vi "Lab Panel V6.00.vi"() -> ()   [LabVIEW 2017] (continued)
                              tunnel: w854 -> [_ _ _ w904 _]
                              tunnel: w853 -> [_ _ _ w914 _]
                              tunnel: w852 -> [_ _ _ w913 _]
                              tunnel: w851 -> [_ _ _ _ _]
                              tunnel: w850 -> [_ _ _ _ w920]
                              frame #0 {
                                w863 = "\\"
                                n604 = case shown="\"CHART TEST\", Default" w876 {
                                tunnel: ["L01-1-CHART TEST-" "L01-1-CYCLE TEST-" "L01-1-T-RISE TEST-"] -> w872
                                frame "CHART TEST", Default {
                                }
                                frame "CYCLE TEST" {
                                }
                                frame "T-RISE TEST" {
                                }
                                }
                                n605 = local read "SET LAB01-1"() -> (w871:T5)
                                n606 = Unbundle By Name(w871) -> ("DESCRIPTION"=w870:string)
                                n607 = Concatenate Strings(w866, "\\", w864, w863, w862, w863) -> (w873:string)
                                n608 = String To Path(string=w873) -> (path=w875:path)
                                n609 = Concatenate Strings(w873, w872, w870, "-", w869, ".tdms") -> (w861:string)
                                n610 = Create Folder(path (use dialog)=w875) -> (error out=w874:errorcluster)  [unwired: 2 in, 2 out]
                                n611 = call <vilib>:"Clear Errors.vi"("error in (no error)"=w874) -> ()  [unwired: 5 in, 2 out]
                                n612 = global write "Global 1.vi" "LAB01-1 FILE"(w861) -> ()
                              }
                              frame #1 {
                                (unwired) FALSE
                                n613 = String To Path(string=w882) -> (path=w880:path)
                                n614 = TDMS Open(6:FALSE, 10:T23."create or replace" ("operation (0:open)"), 11:w880) -> (0:w883:errorcluster, 3:→"TDMS LAB01-1":refnum<k34>)  [unwired: 4 in]
                              }
                              frame #2 {
                                n615 = local read "TDMS LAB01-1"() -> (w902:refnum<k34>)
                                n616 = local read "SET LAB01-1"() -> (w891:T5)
                                n617 = Build Array("Testers Name", "Description", "Set Test Cycles", "T-Rise minutes", "T-Rise Deg C") -> (w892:string[])
                                n618 = Unbundle(w891) -> ("NAME"=w890:string, "DESCRIPTION"=w889:string, "CYCLES"=w888:dbl, "T-RISE mins"=w887:dbl, "T-RISE deg C"=w886:dbl)
                                n619 = Number To Decimal String(number=w888) -> (decimal integer string=w901:string)  [unwired: 1 in]
                                n620 = Number To Decimal String(number=w887) -> (decimal integer string=w900:string)  [unwired: 1 in]
                                n621 = Number To Decimal String(number=w886) -> (decimal integer string=w899:string)  [unwired: 1 in]
                                n622 = Build Array(w890, w889, w901, w900, w899) -> (w898:string[])
                                n623 = TDMS Set Properties(5:w898, 7:w892, 11:w902) -> ()  [unwired: 3 in, 4 out]
                              }
                              frame #3 {
                                n624 = local read "DISP LAB01-1"() -> (w912:T4)
                                n625 = Concatenate Strings("LAB01-1  ", w904) -> (w903:string)
                                n626 = Two Button Dialog(message=w903, 1:w913, 2:w914) -> (T button?=w906:bool)
                                n627 = case shown="True" w906 {
                                tunnel: w912 -> [w917 w918]
                                tunnel: [w917 w918] -> w911
                                tunnel: [w916 w919] -> w910
                                tunnel: [w915 w919] -> w909
                                frame False {
                                n628 = Unbundle(w917) -> ("CYCLE"=w916:dbl, "MINS"=w915:dbl)  [unwired: 1 out]
                                }
                                frame True {
                                w919 = 0.0
                                }
                                }
                                n629 = Bundle(cluster=w911, "CYCLE"=w910, "MINS"=w909, "STATUS"="RUN") -> (w908:T4)
                                n630 = local write "DISP LAB01-1"(w908) -> ()
                              }
                              frame #4 {
                                n631 = local read "TEMP START LAB01-1"() -> (w922:cluster{"TL":dbl, "TN":dbl})
                                n632 = Bundle(cluster=w922, "TL"=w920, "TN"=w920) -> (w921:cluster{"TL":dbl, "TN":dbl})
                                n633 = local write "TEMP START LAB01-1"(w921) -> ()
                              }
                            }
                          }
                        }
                      }
                    }
                  }
                }
              }
              event "RUN LAB01-2": Value Change {
                n634 = event-data() -> ("NewVal"=w927:bool)  [unwired: 1 in, 5 out]
                n635 = local write "run lab01-2"(w927) -> ()
                n636 = case shown="True" w927 {
                  tunnel: w933 -> [_ w971]
                  tunnel: w932 -> [_ w970]
                  tunnel: w930 -> [w935 w969]
                  tunnel: w931 -> [_ w968]
                  tunnel: w929 -> [_ w967]
                  tunnel: [w934 w966] -> w928
                  tunnel: w926 -> [_ w965]
                  tunnel: w925 -> [_ w964]
                  tunnel: w924 -> [_ w963]
                  tunnel: w923 -> [_ w961]
                  frame False {
                    # "stop test"
                    n637 = stacked-sequence {
                      tunnel: w935 -> [w944 _]
                      tunnel: [w936 _] -> w934
                      frame #0 {
                        n638 = local read "DISP LAB01-2"() -> (w943:T4)
                        n639 = Unbundle(w943) -> ("CYCLE"=w941:dbl, "MINS"=w942:dbl)  [unwired: 1 out]
                        n640 = case shown="\"CHART TEST\", Default" w944 {
                          tunnel: w942 -> [_ _ w951]
                          tunnel: w941 -> [w949 w950 _]
                          tunnel: [w949 w950 w951] -> w940
                          frame "CHART TEST", Default {
                          }
                          frame "CYCLE TEST" {
                          }
                          frame "T-RISE TEST" {
                          }
                        }
                        n641 = local read "TDMS LAB01-2"() -> (w948:refnum<k34>)
                        n642 = Build Array("STOPPED") -> (w945:string[])
                        n643 = Build Array(w940) -> (w939:dbl[])
                        n644 = TDMS Write(0:w948, 5:"TEST RESULT", 7:w945, 9:w939) -> (4:w937:refnum<k34>, 15:w938:errorcluster)  [unwired: 2 in, 2 out]
                        n645 = TDMS Close(8:w938, 11:w937) -> (0:w936:errorcluster)  [unwired: 1 out]
                      }
                      frame #1 {
                        n646 = local read "DISP LAB01-2"() -> (w955:T4)
                        n647 = stacked-sequence {
                          tunnel: "LAB01-2" -> [w957 w959]
                          frame #0 {
                            n648 = call "sub vi - defrag tdms v1.vi"("panel id"=w957) -> ("error out"=w956:errorcluster)  [unwired: 10 in]
                            n649 = local write "data file error"(w956) -> ()
                          }
                          frame #1 {
                            n650 = call "Save data file (stop) v3.vi"("panel id"=w959) -> ("network file save error"=w958:errorcluster)  [unwired: 9 in, 1 out]
                            n651 = local write "RESULT LAB01-2"(FALSE) -> ()
                            n652 = local write "data file error"(w958) -> ()
                          }
                        }
                        n653 = Bundle(cluster=w955, "STATUS"="STOP") -> (w953:T4)  [unwired: 2 in]
                        n654 = local write "DISP LAB01-2"(w953) -> ()
                      }
                    }
                  }
                  frame True {
                    n655 = local read "SIG LAB01-2"() -> (w962:T2)
                    n656 = stacked-sequence {
                      seq-local: [w973 _] -> [_ w977]
                      tunnel: w971 -> [_ w987]
                      tunnel: w970 -> [_ w986]
                      tunnel: w969 -> [_ w985]
                      tunnel: w968 -> [_ w984]
                      tunnel: w967 -> [_ w983]
                      tunnel: [_ w982] -> w966
                      tunnel: w965 -> [_ w981]
                      tunnel: w964 -> [_ w980]
                      tunnel: w963 -> [_ w979]
                      tunnel: w962 -> [w972 w978]
                      tunnel: w961 -> [_ w976]
                      frame #0 {
                        n657 = Unbundle(w972) -> ("AMPS"=w975:dbl)  [unwired: 4 out]
                        n658 = call "Check For Amps on v1.vi"("ID"="LAB01-2", "amps"=w975) -> ("amps"=w973:bool)  [unwired: 9 in]
                      }
                      frame #1 {
                        n659 = case shown="True" w977 {
                          tunnel: w987 -> [_ w1000]
                          tunnel: w986 -> [_ w999]
                          tunnel: w985 -> [_ w998]
                          tunnel: w984 -> [_ w997]
                          tunnel: w983 -> [_ w996]
                          tunnel: [errorcluster {"status"=FALSE, "code"=0, "source"=""} ("error out") w995] -> w982
                          tunnel: w981 -> [_ w994]
                          tunnel: w980 -> [_ w993]
                          tunnel: w979 -> [_ w992]
                          tunnel: w978 -> [_ w991]
                          tunnel: w976 -> [_ w990]
                          frame False {
                            w988 = FALSE
                            n660 = local write "RUN LAB01-2"(w988) -> ()
                            n661 = local write "run lab01-2"(w988) -> ()
                          }
                          frame True {
                            n662 = stacked-sequence {
                              seq-local: [w1001 _ _ _ _] -> [_ w1025 _ _ _]
                              tunnel: w1000 -> [w1006 _ _ _ _]
                              tunnel: w999 -> [w1003 _ _ _ _]
                              tunnel: w998 -> [w1016 _ _ _ _]
                              tunnel: w997 -> [w1009 _ _ _ _]
                              tunnel: w996 -> [w1004 _ _ _ _]
                              tunnel: [_ w1020 _ _ _] -> w995
                              tunnel: w994 -> [_ _ _ w1047 _]
                              tunnel: w993 -> [_ _ _ w1046 _]
                              tunnel: w992 -> [_ _ _ w1045 _]
                              tunnel: w991 -> [_ _ _ _ _]
                              tunnel: w990 -> [_ _ _ _ w1060]
                              frame #0 {
                                w1002 = "\\"
                                n663 = local read "SET LAB01-2"() -> (w1011:T5)
                                n664 = case shown="\"CYCLE TEST\"" w1016 {
                                tunnel: ["L01-2-CHART TEST-" "L01-2-CYCLE TEST-" "L01-2-T-RISE TEST-"] -> w1012
                                frame "CHART TEST", Default {
                                }
                                frame "CYCLE TEST" {
                                }
                                frame "T-RISE TEST" {
                                }
                                }
                                n665 = Unbundle(w1011) -> ("DESCRIPTION"=w1010:string)  [unwired: 4 out]
                                n666 = Concatenate Strings(w1006, "\\", w1004, w1002, w1003, w1002) -> (w1013:string)
                                n667 = String To Path(string=w1013) -> (path=w1015:path)
                                n668 = Concatenate Strings(w1013, w1012, w1010, "-", w1009, ".tdms") -> (w1001:string)
                                n669 = Create Folder(path (use dialog)=w1015) -> (error out=w1014:errorcluster)  [unwired: 2 in, 2 out]
                                n670 = call <vilib>:"Clear Errors.vi"("error in (no error)"=w1014) -> ()  [unwired: 5 in, 2 out]
                                n671 = global write "Global 1.vi" "LAB01-2 FILE"(w1001) -> ()
                              }
                              frame #1 {
                                (unwired) FALSE
                                n672 = String To Path(string=w1025) -> (path=w1021:path)
                                n673 = TDMS Open(6:FALSE, 10:T23."create or replace" ("operation (0:open)"), 11:w1021) -> (0:w1020:errorcluster, 3:→"TDMS LAB01-2":refnum<k34>)  [unwired: 4 in]
                              }
                              frame #2 {
                                n674 = local read "SET LAB01-2"() -> (w1031:T5)
                                n675 = local read "TDMS LAB01-2"() -> (w1042:refnum<k34>)
                                n676 = Build Array("Testers Name", "Description", "Set Test Cycles", "T-Rise minutes", "T-Rise Deg C") -> (w1032:string[])
                                n677 = Unbundle(w1031) -> ("NAME"=w1030:string, "DESCRIPTION"=w1029:string, "CYCLES"=w1028:dbl, "T-RISE mins"=w1027:dbl, "T-RISE deg C"=w1026:dbl)
                                n678 = Number To Decimal String(number=w1028) -> (decimal integer string=w1041:string)  [unwired: 1 in]
                                n679 = Number To Decimal String(number=w1027) -> (decimal integer string=w1040:string)  [unwired: 1 in]
                                n680 = Number To Decimal String(number=w1026) -> (decimal integer string=w1039:string)  [unwired: 1 in]
                                n681 = Build Array(w1030, w1029, w1041, w1040, w1039) -> (w1038:string[])
                                n682 = TDMS Set Properties(5:w1038, 7:w1032, 11:w1042) -> ()  [unwired: 3 in, 4 out]
                              }
                              frame #3 {
                                n683 = local read "DISP LAB01-2"() -> (w1044:T4)
                                n684 = Concatenate Strings("LAB01-2  ", w1047) -> (w1048:string)
                                n685 = Two Button Dialog(message=w1048, 1:w1045, 2:w1046) -> (T button?=w1050:bool)
                                n686 = case shown="True" w1050 {
                                tunnel: w1044 -> [w1057 w1058]
                                tunnel: [w1057 w1058] -> w1054
                                tunnel: [w1056 w1059] -> w1053
                                tunnel: [w1055 w1059] -> w1052
                                frame False {
                                n687 = Unbundle(w1057) -> ("CYCLE"=w1056:dbl, "MINS"=w1055:dbl)  [unwired: 1 out]
                                }
                                frame True {
                                w1059 = 0.0
                                }
                                }
                                n688 = Bundle(cluster=w1054, "CYCLE"=w1053, "MINS"=w1052, "STATUS"="RUN") -> (w1043:T4)
                                n689 = local write "DISP LAB01-2"(w1043) -> ()
                              }
                              frame #4 {
                                n690 = local read "TEMP START LAB01-2"() -> (w1062:cluster{"TL":dbl, "TN":dbl})
                                n691 = Bundle(cluster=w1062, "TL"=w1060, "TN"=w1060) -> (w1061:cluster{"TL":dbl, "TN":dbl})
                                n692 = local write "TEMP START LAB01-2"(w1061) -> ()
                              }
                            }
                          }
                        }
                      }
                    }
                  }
                }
              }
              event "RUN LAB02-1": Value Change {
                n693 = event-data() -> ("NewVal"=w1068:bool)  [unwired: 1 in, 5 out]
                n694 = local read "SIG LAB02-1"() -> (w1064:T2)
                n695 = case shown="True" w1068 {
                  tunnel: w1074 -> [_ w1112]
                  tunnel: w1073 -> [_ w1111]
                  tunnel: w1071 -> [w1076 w1110]
                  tunnel: w1072 -> [_ w1109]
                  tunnel: w1070 -> [_ w1108]
                  tunnel: [w1075 w1107] -> w1069
                  tunnel: w1067 -> [_ w1106]
                  tunnel: w1066 -> [_ w1105]
                  tunnel: w1065 -> [_ w1104]
                  tunnel: w1064 -> [_ w1103]
                  tunnel: w1063 -> [_ w1102]
                  frame False {
                    # "stop test"
                    n696 = stacked-sequence {
                      tunnel: w1076 -> [w1085 _]
                      tunnel: [w1077 _] -> w1075
                      frame #0 {
                        n697 = local read "DISP LAB02-1"() -> (w1084:T4)
                        n698 = Unbundle(w1084) -> ("CYCLE"=w1082:dbl, "MINS"=w1083:dbl)  [unwired: 1 out]
                        n699 = case shown="\"CYCLE TEST\"" w1085 {
                          tunnel: w1083 -> [_ _ w1092]
                          tunnel: w1082 -> [w1090 w1091 _]
                          tunnel: [w1090 w1091 w1092] -> w1081
                          frame "CHART TEST", Default {
                          }
                          frame "CYCLE TEST" {
                          }
                          frame "T-RISE TEST" {
                          }
                        }
                        n700 = local read "TDMS LAB02-1"() -> (w1089:refnum<k34>)
                        n701 = Build Array("STOPPED") -> (w1086:string[])
                        n702 = Build Array(w1081) -> (w1080:dbl[])
                        n703 = TDMS Write(0:w1089, 5:"TEST RESULT", 7:w1086, 9:w1080) -> (4:w1078:refnum<k34>, 15:w1079:errorcluster)  [unwired: 2 in, 2 out]
                        n704 = TDMS Close(8:w1079, 11:w1078) -> (0:w1077:errorcluster)  [unwired: 1 out]
                      }
                      frame #1 {
                        n705 = local read "DISP LAB02-1"() -> (w1096:T4)
                        n706 = stacked-sequence {
                          tunnel: "LAB02-1" -> [w1098 w1100]
                          frame #0 {
                            n707 = call "sub vi - defrag tdms v1.vi"("panel id"=w1098) -> ("error out"=w1097:errorcluster)  [unwired: 10 in]
                            n708 = local write "data file error"(w1097) -> ()
                          }
                          frame #1 {
                            n709 = local write "RESULT LAB02-1"(FALSE) -> ()
                            n710 = call "Save data file (stop) v3.vi"("panel id"=w1100) -> ("network file save error"=w1099:errorcluster)  [unwired: 9 in, 1 out]
                            n711 = local write "data file error"(w1099) -> ()
                          }
                        }
                        n712 = Bundle(cluster=w1096, "STATUS"="STOP") -> (w1094:T4)  [unwired: 2 in]
                        n713 = local write "DISP LAB02-1"(w1094) -> ()
                      }
                    }
                  }
                  frame True {
                    n714 = stacked-sequence {
                      seq-local: [w1114 _] -> [_ w1118]
                      tunnel: w1112 -> [_ w1128]
                      tunnel: w1111 -> [_ w1127]
                      tunnel: w1110 -> [_ w1126]
                      tunnel: w1109 -> [_ w1125]
                      tunnel: w1108 -> [_ w1124]
                      tunnel: [_ w1123] -> w1107
                      tunnel: w1106 -> [_ w1122]
                      tunnel: w1105 -> [_ w1121]
                      tunnel: w1104 -> [_ w1120]
                      tunnel: w1103 -> [w1113 w1119]
                      tunnel: w1102 -> [_ w1117]
                      frame #0 {
                        n715 = Unbundle(w1113) -> ("AMPS"=w1116:dbl)  [unwired: 4 out]
                        n716 = call "Check For Amps on v1.vi"("ID"="LAB02-1", "amps"=w1116) -> ("amps"=w1114:bool)  [unwired: 9 in]
                      }
                      frame #1 {
                        n717 = case shown="True" w1118 {
                          tunnel: w1128 -> [_ w1141]
                          tunnel: w1127 -> [_ w1140]
                          tunnel: w1126 -> [_ w1139]
                          tunnel: w1125 -> [_ w1138]
                          tunnel: w1124 -> [_ w1137]
                          tunnel: [errorcluster {"status"=FALSE, "code"=0, "source"=""} ("error out") w1136] -> w1123
                          tunnel: w1122 -> [_ w1135]
                          tunnel: w1121 -> [_ w1134]
                          tunnel: w1120 -> [_ w1133]
                          tunnel: w1119 -> [_ w1132]
                          tunnel: w1117 -> [_ w1131]
                          frame False {
                            w1130 = FALSE
                            n718 = local write "RUN LAB02-1"(w1130) -> ()
                            n719 = local write "run lab02-1"(w1130) -> ()
                          }
                          frame True {
                            n720 = stacked-sequence {
                              seq-local: [w1142 _ _ _ _] -> [_ w1166 _ _ _]
                              tunnel: w1141 -> [w1147 _ _ _ _]
                              tunnel: w1140 -> [w1144 _ _ _ _]
                              tunnel: w1139 -> [w1157 _ _ _ _]
                              tunnel: w1138 -> [w1150 _ _ _ _]
                              tunnel: w1137 -> [w1145 _ _ _ _]
                              tunnel: [_ w1161 _ _ _] -> w1136
                              tunnel: w1135 -> [_ _ _ w1187 _]
                              tunnel: w1134 -> [_ _ _ w1186 _]
                              tunnel: w1133 -> [_ _ _ w1185 _]
                              tunnel: w1132 -> [_ _ _ _ _]
                              tunnel: w1131 -> [_ _ _ _ w1201]
                              frame #0 {
                                w1143 = "\\"
                                n721 = local read "SET LAB02-1"() -> (w1152:T5)
                                n722 = case shown="\"CYCLE TEST\"" w1157 {
                                tunnel: ["L02-1-CHART TEST-" "L02-1-CYCLE TEST-" "L02-1-T-RISE TEST-"] -> w1153
                                frame "CHART TEST", Default {
                                }
                                frame "CYCLE TEST" {
                                }
                                frame "T-RISE TEST" {
                                }
                                }
                                n723 = Unbundle(w1152) -> ("DESCRIPTION"=w1151:string)  [unwired: 4 out]
                                n724 = Concatenate Strings(w1147, "\\", w1145, w1143, w1144, w1143) -> (w1154:string)
                                n725 = String To Path(string=w1154) -> (path=w1156:path)
                                n726 = Concatenate Strings(w1154, w1153, w1151, "-", w1150, ".tdms") -> (w1142:string)
                                n727 = Create Folder(path (use dialog)=w1156) -> (error out=w1155:errorcluster)  [unwired: 2 in, 2 out]
                                n728 = global write "Global 1.vi" "LAB02-1 FILE"(w1142) -> ()
                                n729 = call <vilib>:"Clear Errors.vi"("error in (no error)"=w1155) -> ()  [unwired: 5 in, 2 out]
                              }
                              frame #1 {
                                (unwired) FALSE
                                n730 = String To Path(string=w1166) -> (path=w1162:path)
                                n731 = TDMS Open(6:FALSE, 10:T23."create or replace" ("operation (0:open)"), 11:w1162) -> (0:w1161:errorcluster, 3:→"TDMS LAB02-1":refnum<k34>)  [unwired: 4 in]
                              }
                              frame #2 {
                                n732 = local read "SET LAB02-1"() -> (w1172:T5)
                                n733 = local read "TDMS LAB02-1"() -> (w1183:refnum<k34>)
                                n734 = Build Array("Testers Name", "Description", "Set Test Cycles", "T-Rise minutes", "T-Rise Deg C") -> (w1173:string[])
                                n735 = Unbundle(w1172) -> ("NAME"=w1171:string, "DESCRIPTION"=w1170:string, "CYCLES"=w1169:dbl, "T-RISE mins"=w1168:dbl, "T-RISE deg C"=w1167:dbl)
                                n736 = Number To Decimal String(number=w1169) -> (decimal integer string=w1182:string)  [unwired: 1 in]
                                n737 = Number To Decimal String(number=w1168) -> (decimal integer string=w1181:string)  [unwired: 1 in]
                                n738 = Number To Decimal String(number=w1167) -> (decimal integer string=w1180:string)  [unwired: 1 in]
                                n739 = Build Array(w1171, w1170, w1182, w1181, w1180) -> (w1179:string[])
                                n740 = TDMS Set Properties(5:w1179, 7:w1173, 11:w1183) -> ()  [unwired: 3 in, 4 out]
                              }
                              frame #3 {
                                n741 = local read "DISP LAB02-1"() -> (w1188:T4)
                                n742 = Concatenate Strings("LAB02-1  ", w1187) -> (w1189:string)
                                n743 = Two Button Dialog(message=w1189, 1:w1185, 2:w1186) -> (T button?=w1191:bool)
                                n744 = case shown="True" w1191 {
                                tunnel: w1188 -> [w1198 w1199]
                                tunnel: [w1198 w1199] -> w1195
                                tunnel: [w1197 w1200] -> w1194
                                tunnel: [w1196 w1200] -> w1193
                                frame False {
                                n745 = Unbundle(w1198) -> ("CYCLE"=w1197:dbl, "MINS"=w1196:dbl)  [unwired: 1 out]
                                }
                                frame True {
                                w1200 = 0.0
                                }
                                }
                                n746 = Bundle(cluster=w1195, "CYCLE"=w1194, "MINS"=w1193, "STATUS"="RUN") -> (w1184:T4)
                                n747 = local write "DISP LAB02-1"(w1184) -> ()
                              }
                              frame #4 {
                                n748 = local read "TEMP START LAB02-1"() -> (w1203:cluster{"TL":dbl, "TN":dbl})
                                n749 = Bundle(cluster=w1203, "TL"=w1201, "TN"=w1201) -> (w1202:cluster{"TL":dbl, "TN":dbl})
                                n750 = local write "TEMP START LAB02-1"(w1202) -> ()
                              }
                            }
                          }
                        }
                      }
                    }
                  }
                }
                n751 = local write "run lab02-1"(w1068) -> ()
              }
              event "RUN LAB02-2": Value Change {
                n752 = event-data() -> ("NewVal"=w1208:bool)  [unwired: 1 in, 5 out]
                n753 = local write "run lab02-2"(w1208) -> ()
                n754 = case shown="True" w1208 {
                  tunnel: w1214 -> [_ w1252]
                  tunnel: w1213 -> [_ w1251]
                  tunnel: w1211 -> [w1216 w1250]
                  tunnel: w1212 -> [_ w1249]
                  tunnel: w1210 -> [_ w1248]
                  tunnel: [w1215 w1247] -> w1209
                  tunnel: w1207 -> [_ w1246]
                  tunnel: w1206 -> [_ w1245]
                  tunnel: w1205 -> [_ w1244]
                  tunnel: w1204 -> [_ w1242]
                  frame False {
                    # "stop test"
                    n755 = stacked-sequence {
                      tunnel: w1216 -> [w1225 _]
                      tunnel: [w1217 _] -> w1215
                      frame #0 {
                        n756 = local read "DISP LAB02-2"() -> (w1224:T4)
                        n757 = Unbundle(w1224) -> ("CYCLE"=w1222:dbl, "MINS"=w1223:dbl)  [unwired: 1 out]
                        n758 = case shown="\"CYCLE TEST\"" w1225 {
                          tunnel: w1223 -> [_ _ w1232]
                          tunnel: w1222 -> [w1230 w1231 _]
                          tunnel: [w1230 w1231 w1232] -> w1221
                          frame "CHART TEST", Default {
                          }
                          frame "CYCLE TEST" {
                          }
                          frame "T-RISE TEST" {
                          }
                        }
                        n759 = local read "TDMS LAB02-2"() -> (w1229:refnum<k34>)
                        n760 = Build Array("STOPPED") -> (w1226:string[])
                        n761 = Build Array(w1221) -> (w1220:dbl[])
                        n762 = TDMS Write(0:w1229, 5:"TEST RESULT", 7:w1226, 9:w1220) -> (4:w1218:refnum<k34>, 15:w1219:errorcluster)  [unwired: 2 in, 2 out]
                        n763 = TDMS Close(8:w1219, 11:w1218) -> (0:w1217:errorcluster)  [unwired: 1 out]
                      }
                      frame #1 {
                        n764 = local read "DISP LAB02-2"() -> (w1236:T4)
                        n765 = stacked-sequence {
                          tunnel: "LAB02-2" -> [w1238 w1240]
                          frame #0 {
                            n766 = call "sub vi - defrag tdms v1.vi"("panel id"=w1238) -> ("error out"=w1237:errorcluster)  [unwired: 10 in]
                            n767 = local write "data file error"(w1237) -> ()
                          }
                          frame #1 {
                            n768 = call "Save data file (stop) v3.vi"("panel id"=w1240) -> ("network file save error"=w1239:errorcluster)  [unwired: 9 in, 1 out]
                            n769 = local write "RESULT LAB02-2"(FALSE) -> ()
                            n770 = local write "data file error"(w1239) -> ()
                          }
                        }
                        n771 = Bundle(cluster=w1236, "STATUS"="STOP") -> (w1234:T4)  [unwired: 2 in]
                        n772 = local write "DISP LAB02-2"(w1234) -> ()
                      }
                    }
                  }
                  frame True {
                    n773 = local read "SIG LAB02-2"() -> (w1243:T2)
                    n774 = stacked-sequence {
                      seq-local: [w1254 _] -> [_ w1258]
                      tunnel: w1252 -> [_ w1268]
                      tunnel: w1251 -> [_ w1267]
                      tunnel: w1250 -> [_ w1266]
                      tunnel: w1249 -> [_ w1265]
                      tunnel: w1248 -> [_ w1264]
                      tunnel: [_ w1263] -> w1247
                      tunnel: w1246 -> [_ w1262]
                      tunnel: w1245 -> [_ w1261]
                      tunnel: w1244 -> [_ w1260]
                      tunnel: w1243 -> [w1253 w1259]
                      tunnel: w1242 -> [_ w1257]
                      frame #0 {
                        n775 = Unbundle(w1253) -> ("AMPS"=w1256:dbl)  [unwired: 4 out]
                        n776 = call "Check For Amps on v1.vi"("ID"="LAB02-2", "amps"=w1256) -> ("amps"=w1254:bool)  [unwired: 9 in]
                      }
                      frame #1 {
                        n777 = case shown="True" w1258 {
                          tunnel: w1268 -> [_ w1281]
                          tunnel: w1267 -> [_ w1280]
                          tunnel: w1266 -> [_ w1279]
                          tunnel: w1265 -> [_ w1278]
                          tunnel: w1264 -> [_ w1277]
                          tunnel: [errorcluster {"status"=FALSE, "code"=0, "source"=""} ("error out") w1276] -> w1263
                          tunnel: w1262 -> [_ w1275]
                          tunnel: w1261 -> [_ w1274]
                          tunnel: w1260 -> [_ w1273]
                          tunnel: w1259 -> [_ w1272]
                          tunnel: w1257 -> [_ w1271]
                          frame False {
                            w1269 = FALSE
                            n778 = local write "RUN LAB02-2"(w1269) -> ()
                            n779 = local write "run lab02-2"(w1269) -> ()
                          }
                          frame True {
                            n780 = stacked-sequence {
                              seq-local: [w1282 _ _ _ _] -> [_ w1306 _ _ _]
                              tunnel: w1281 -> [w1287 _ _ _ _]
                              tunnel: w1280 -> [w1284 _ _ _ _]
                              tunnel: w1279 -> [w1297 _ _ _ _]
                              tunnel: w1278 -> [w1290 _ _ _ _]
                              tunnel: w1277 -> [w1285 _ _ _ _]
                              tunnel: [_ w1301 _ _ _] -> w1276
                              tunnel: w1275 -> [_ _ _ w1327 _]
                              tunnel: w1274 -> [_ _ _ w1326 _]
                              tunnel: w1273 -> [_ _ _ w1325 _]
                              tunnel: w1272 -> [_ _ _ _ _]
                              tunnel: w1271 -> [_ _ _ _ w1341]
                              frame #0 {
                                w1283 = "\\"
                                n781 = local read "SET LAB02-2"() -> (w1292:T5)
                                n782 = case shown="\"CYCLE TEST\"" w1297 {
                                tunnel: ["L02-2-CHART TEST-" "L02-2-CYCLE TEST-" "L02-2-T-RISE TEST-"] -> w1293
                                frame "CHART TEST", Default {
                                }
                                frame "CYCLE TEST" {
                                }
                                frame "T-RISE TEST" {
                                }
                                }
                                n783 = Unbundle(w1292) -> ("DESCRIPTION"=w1291:string)  [unwired: 4 out]
                                n784 = Concatenate Strings(w1287, "\\", w1285, w1283, w1284, w1283) -> (w1294:string)
                                n785 = String To Path(string=w1294) -> (path=w1296:path)
                                n786 = Concatenate Strings(w1294, w1293, w1291, "-", w1290, ".tdms") -> (w1282:string)
                                n787 = Create Folder(path (use dialog)=w1296) -> (error out=w1295:errorcluster)  [unwired: 2 in, 2 out]
                                n788 = global write "Global 1.vi" "LAB02-2 FILE"(w1282) -> ()
                                n789 = call <vilib>:"Clear Errors.vi"("error in (no error)"=w1295) -> ()  [unwired: 5 in, 2 out]
                              }
                              frame #1 {
                                (unwired) FALSE
                                n790 = String To Path(string=w1306) -> (path=w1302:path)
                                n791 = TDMS Open(6:FALSE, 10:T23."create or replace" ("operation (0:open)"), 11:w1302) -> (0:w1301:errorcluster, 3:→"TDMS LAB02-2":refnum<k34>)  [unwired: 4 in]
                              }
                              frame #2 {
                                n792 = local read "SET LAB02-2"() -> (w1312:T5)
                                n793 = local read "TDMS LAB02-2"() -> (w1323:refnum<k34>)
                                n794 = Build Array("Testers Name", "Description", "Set Test Cycles", "T-Rise minutes", "T-Rise Deg C") -> (w1313:string[])
                                n795 = Unbundle(w1312) -> ("NAME"=w1311:string, "DESCRIPTION"=w1310:string, "CYCLES"=w1309:dbl, "T-RISE mins"=w1308:dbl, "T-RISE deg C"=w1307:dbl)
                                n796 = Number To Decimal String(number=w1309) -> (decimal integer string=w1322:string)  [unwired: 1 in]
                                n797 = Number To Decimal String(number=w1308) -> (decimal integer string=w1321:string)  [unwired: 1 in]
                                n798 = Number To Decimal String(number=w1307) -> (decimal integer string=w1320:string)  [unwired: 1 in]
                                n799 = Build Array(w1311, w1310, w1322, w1321, w1320) -> (w1319:string[])
                                n800 = TDMS Set Properties(5:w1319, 7:w1313, 11:w1323) -> ()  [unwired: 3 in, 4 out]
                              }
                              frame #3 {
                                n801 = local read "DISP LAB02-2"() -> (w1328:T4)
                                n802 = Concatenate Strings("LAB02-2  ", w1327) -> (w1329:string)
                                n803 = Two Button Dialog(message=w1329, 1:w1325, 2:w1326) -> (T button?=w1331:bool)
                                n804 = case shown="True" w1331 {
                                tunnel: w1328 -> [w1338 w1339]
                                tunnel: [w1338 w1339] -> w1335
                                tunnel: [w1337 w1340] -> w1334
                                tunnel: [w1336 w1340] -> w1333
                                frame False {
                                n805 = Unbundle(w1338) -> ("CYCLE"=w1337:dbl, "MINS"=w1336:dbl)  [unwired: 1 out]
                                }
                                frame True {
                                w1340 = 0.0
                                }
                                }
                                n806 = Bundle(cluster=w1335, "CYCLE"=w1334, "MINS"=w1333, "STATUS"="RUN") -> (w1324:T4)
                                n807 = local write "DISP LAB02-2"(w1324) -> ()
                              }
                              frame #4 {
                                n808 = local read "TEMP START LAB02-2"() -> (w1343:cluster{"TL":dbl, "TN":dbl})
                                n809 = Bundle(cluster=w1343, "TL"=w1341, "TN"=w1341) -> (w1342:cluster{"TL":dbl, "TN":dbl})
                                n810 = local write "TEMP START LAB02-2"(w1342) -> ()
                              }
                            }
                          }
                        }
                      }
                    }
                  }
                }
              }
              event "RUN LAB03-1": Value Change {
                n811 = event-data() -> ("NewVal"=w1348:bool)  [unwired: 1 in, 5 out]
                n812 = local write "run lab03-1"(w1348) -> ()
                n813 = case shown="True" w1348 {
                  tunnel: w1354 -> [_ w1392]
                  tunnel: w1353 -> [_ w1391]
                  tunnel: w1351 -> [w1356 w1390]
                  tunnel: w1352 -> [_ w1389]
                  tunnel: w1350 -> [_ w1388]
                  tunnel: [w1355 w1387] -> w1349
                  tunnel: w1347 -> [_ w1386]
                  tunnel: w1346 -> [_ w1385]
                  tunnel: w1345 -> [_ w1384]
                  tunnel: w1344 -> [_ w1382]
                  frame False {
                    # "stop test"
                    n814 = stacked-sequence {
                      tunnel: w1356 -> [w1365 _]
                      tunnel: [w1357 _] -> w1355
                      frame #0 {
                        n815 = local read "DISP LAB03-1"() -> (w1364:T4)
                        n816 = Unbundle(w1364) -> ("CYCLE"=w1362:dbl, "MINS"=w1363:dbl)  [unwired: 1 out]
                        n817 = case shown="\"CYCLE TEST\"" w1365 {
                          tunnel: w1363 -> [_ _ w1372]
                          tunnel: w1362 -> [w1370 w1371 _]
                          tunnel: [w1370 w1371 w1372] -> w1361
                          frame "CHART TEST", Default {
                          }
                          frame "CYCLE TEST" {
                          }
                          frame "T-RISE TEST" {
                          }
                        }
                        n818 = local read "TDMS LAB03-1"() -> (w1369:refnum<k34>)
                        n819 = Build Array("STOPPED") -> (w1366:string[])
                        n820 = Build Array(w1361) -> (w1360:dbl[])
                        n821 = TDMS Write(0:w1369, 5:"TEST RESULT", 7:w1366, 9:w1360) -> (4:w1358:refnum<k34>, 15:w1359:errorcluster)  [unwired: 2 in, 2 out]
                        n822 = TDMS Close(8:w1359, 11:w1358) -> (0:w1357:errorcluster)  [unwired: 1 out]
                      }
                      frame #1 {
                        n823 = local read "DISP LAB03-1"() -> (w1376:T4)
                        n824 = stacked-sequence {
                          tunnel: "LAB03-1" -> [w1378 w1380]
                          frame #0 {
                            n825 = call "sub vi - defrag tdms v1.vi"("panel id"=w1378) -> ("error out"=w1377:errorcluster)  [unwired: 10 in]
                            n826 = local write "data file error"(w1377) -> ()
                          }
                          frame #1 {
                            n827 = call "Save data file (stop) v3.vi"("panel id"=w1380) -> ("network file save error"=w1379:errorcluster)  [unwired: 9 in, 1 out]
                            n828 = local write "RESULT LAB03-1"(FALSE) -> ()
                            n829 = local write "data file error"(w1379) -> ()
                          }
                        }
                        n830 = Bundle(cluster=w1376, "STATUS"="STOP") -> (w1374:T4)  [unwired: 2 in]
                        n831 = local write "DISP LAB03-1"(w1374) -> ()
                      }
                    }
                  }
                  frame True {
                    n832 = local read "SIG LAB03-1"() -> (w1383:T2)
                    n833 = stacked-sequence {
                      seq-local: [w1394 _] -> [_ w1398]
                      tunnel: w1392 -> [_ w1408]
                      tunnel: w1391 -> [_ w1407]
                      tunnel: w1390 -> [_ w1406]
                      tunnel: w1389 -> [_ w1405]
                      tunnel: w1388 -> [_ w1404]
                      tunnel: [_ w1403] -> w1387
                      tunnel: w1386 -> [_ w1402]
                      tunnel: w1385 -> [_ w1401]
                      tunnel: w1384 -> [_ w1400]
                      tunnel: w1383 -> [w1393 w1399]
                      tunnel: w1382 -> [_ w1397]
                      frame #0 {
                        n834 = Unbundle(w1393) -> ("AMPS"=w1396:dbl)  [unwired: 4 out]
                        n835 = call "Check For Amps on v1.vi"("ID"="LAB03-1", "amps"=w1396) -> ("amps"=w1394:bool)  [unwired: 9 in]
                      }
                      frame #1 {
                        n836 = case shown="True" w1398 {
                          tunnel: w1408 -> [_ w1421]
                          tunnel: w1407 -> [_ w1420]
                          tunnel: w1406 -> [_ w1419]
                          tunnel: w1405 -> [_ w1418]
                          tunnel: w1404 -> [_ w1417]
                          tunnel: [errorcluster {"status"=FALSE, "code"=0, "source"=""} ("error out") w1416] -> w1403
                          tunnel: w1402 -> [_ w1415]
                          tunnel: w1401 -> [_ w1414]
                          tunnel: w1400 -> [_ w1413]
                          tunnel: w1399 -> [_ w1412]
                          tunnel: w1397 -> [_ w1411]
                          frame False {
                            w1409 = FALSE
                            n837 = local write "RUN LAB03-1"(w1409) -> ()
                            n838 = local write "run lab03-1"(w1409) -> ()
                          }
                          frame True {
                            n839 = stacked-sequence {
                              seq-local: [w1422 _ _ _ _] -> [_ w1446 _ _ _]
                              tunnel: w1421 -> [w1427 _ _ _ _]
                              tunnel: w1420 -> [w1424 _ _ _ _]
                              tunnel: w1419 -> [w1437 _ _ _ _]
                              tunnel: w1418 -> [w1430 _ _ _ _]
                              tunnel: w1417 -> [w1425 _ _ _ _]
                              tunnel: [_ w1441 _ _ _] -> w1416
                              tunnel: w1415 -> [_ _ _ w1466 _]
                              tunnel: w1414 -> [_ _ _ w1465 _]
                              tunnel: w1413 -> [_ _ _ w1464 _]
                              tunnel: w1412 -> [_ _ _ _ _]
                              tunnel: w1411 -> [_ _ _ _ w1481]
                              frame #0 {
                                w1423 = "\\"
                                n840 = local read "SET LAB03-1"() -> (w1432:T5)
                                n841 = case shown="\"T-RISE TEST\"" w1437 {
                                tunnel: ["L03-1-CHART TEST-" "L03-1-CYCLE TEST-" "L03-1-T-RISE TEST-"] -> w1433
                                frame "CHART TEST", Default {
                                }
                                frame "CYCLE TEST" {
                                }
                                frame "T-RISE TEST" {
                                }
                                }
                                n842 = Unbundle(w1432) -> ("DESCRIPTION"=w1431:string)  [unwired: 4 out]
                                n843 = Concatenate Strings(w1427, "\\", w1425, w1423, w1424, w1423) -> (w1434:string)
                                n844 = String To Path(string=w1434) -> (path=w1436:path)
                                n845 = Concatenate Strings(w1434, w1433, w1431, "-", w1430, ".tdms") -> (w1422:string)
                                n846 = Create Folder(path (use dialog)=w1436) -> (error out=w1435:errorcluster)  [unwired: 2 in, 2 out]
                                n847 = global write "Global 1.vi" "LAB03-1 FILE"(w1422) -> ()
                                n848 = call <vilib>:"Clear Errors.vi"("error in (no error)"=w1435) -> ()  [unwired: 5 in, 2 out]
                              }
                              frame #1 {
                                (unwired) FALSE
                                n849 = String To Path(string=w1446) -> (path=w1442:path)
                                n850 = TDMS Open(6:FALSE, 10:T23."create or replace" ("operation (0:open)"), 11:w1442) -> (0:w1441:errorcluster, 3:→"TDMS LAB03-1":refnum<k34>)  [unwired: 4 in]
                              }
                              frame #2 {
                                n851 = local read "SET LAB03-1"() -> (w1452:T5)
                                n852 = local read "TDMS LAB03-1"() -> (w1463:refnum<k34>)
                                n853 = Build Array("Testers Name", "Description", "Set Test Cycles", "T-Rise minutes", "T-Rise Deg C") -> (w1453:string[])
                                n854 = Unbundle(w1452) -> ("NAME"=w1451:string, "DESCRIPTION"=w1450:string, "CYCLES"=w1449:dbl, "T-RISE mins"=w1448:dbl, "T-RISE deg C"=w1447:dbl)
                                n855 = Number To Decimal String(number=w1449) -> (decimal integer string=w1462:string)  [unwired: 1 in]
                                n856 = Number To Decimal String(number=w1448) -> (decimal integer string=w1461:string)  [unwired: 1 in]
                                n857 = Number To Decimal String(number=w1447) -> (decimal integer string=w1460:string)  [unwired: 1 in]
                                n858 = Build Array(w1451, w1450, w1462, w1461, w1460) -> (w1459:string[])
                                n859 = TDMS Set Properties(5:w1459, 7:w1453, 11:w1463) -> ()  [unwired: 3 in, 4 out]
                              }
                              frame #3 {
                                n860 = local read "DISP LAB03-1"() -> (w1468:T4)
                                n861 = Concatenate Strings("LAB03-1  ", w1466) -> (w1469:string)
                                n862 = Two Button Dialog(message=w1469, 1:w1464, 2:w1465) -> (T button?=w1471:bool)
                                n863 = case shown="True" w1471 {
                                tunnel: w1468 -> [w1478 w1479]
                                tunnel: [w1478 w1479] -> w1475
                                tunnel: [w1477 w1480] -> w1474
                                tunnel: [w1476 w1480] -> w1473
                                frame False {
                                n864 = Unbundle(w1478) -> ("CYCLE"=w1477:dbl, "MINS"=w1476:dbl)  [unwired: 1 out]
                                }
                                frame True {
                                w1480 = 0.0
                                }
                                }
                                n865 = Bundle(cluster=w1475, "CYCLE"=w1474, "MINS"=w1473, "STATUS"="RUN") -> (w1467:T4)
                                n866 = local write "DISP LAB03-1"(w1467) -> ()
                              }
                              frame #4 {
                                n867 = local read "TEMP START LAB03-1"() -> (w1483:cluster{"TL":dbl, "TN":dbl})
                                n868 = Bundle(cluster=w1483, "TL"=w1481, "TN"=w1481) -> (w1482:cluster{"TL":dbl, "TN":dbl})
                                n869 = local write "TEMP START LAB03-1"(w1482) -> ()
                              }
                            }
                          }
                        }
                      }
                    }
                  }
                }
              }
              event "RUN LAB03-2": Value Change {
                n870 = event-data() -> ("NewVal"=w1488:bool)  [unwired: 1 in, 5 out]
                n871 = local write "run lab03-2"(w1488) -> ()
                n872 = case shown="True" w1488 {
                  tunnel: w1494 -> [_ w1532]
                  tunnel: w1493 -> [_ w1531]
                  tunnel: w1491 -> [w1496 w1530]
                  tunnel: w1492 -> [_ w1529]
                  tunnel: w1490 -> [_ w1528]
                  tunnel: [w1495 w1527] -> w1489
                  tunnel: w1487 -> [_ w1526]
                  tunnel: w1486 -> [_ w1525]
                  tunnel: w1485 -> [_ w1524]
                  tunnel: w1484 -> [_ w1522]
                  frame False {
                    # "stop test"
                    n873 = stacked-sequence {
                      tunnel: w1496 -> [w1505 _]
                      tunnel: [w1497 _] -> w1495
                      frame #0 {
                        n874 = local read "DISP LAB03-2"() -> (w1504:T4)
                        n875 = Unbundle(w1504) -> ("CYCLE"=w1502:dbl, "MINS"=w1503:dbl)  [unwired: 1 out]
                        n876 = case shown="\"CYCLE TEST\"" w1505 {
                          tunnel: w1503 -> [_ _ w1512]
                          tunnel: w1502 -> [w1510 w1511 _]
                          tunnel: [w1510 w1511 w1512] -> w1501
